vi "Router - Reader.vi"(8 "error in (no error)":errorcluster, 11 "Router Data In":T1) -> (0 "error out":errorcluster, 3 "Router Data Out":T1)   [LabVIEW 2016, in "PXImc Router.lvlib"]
uses:
  PXImc Router.lvlib
  Controls/Router - Configuration.ctl
  Controls/Target Type.ctl
  Controls/Router/Node Block R-W Properties.ctl
  Controls/Router/Block Properties.ctl
  Controls/Router/Router - PXImc Properties.ctl
  Controls/Router/Router - PXImc Card Properties.ctl
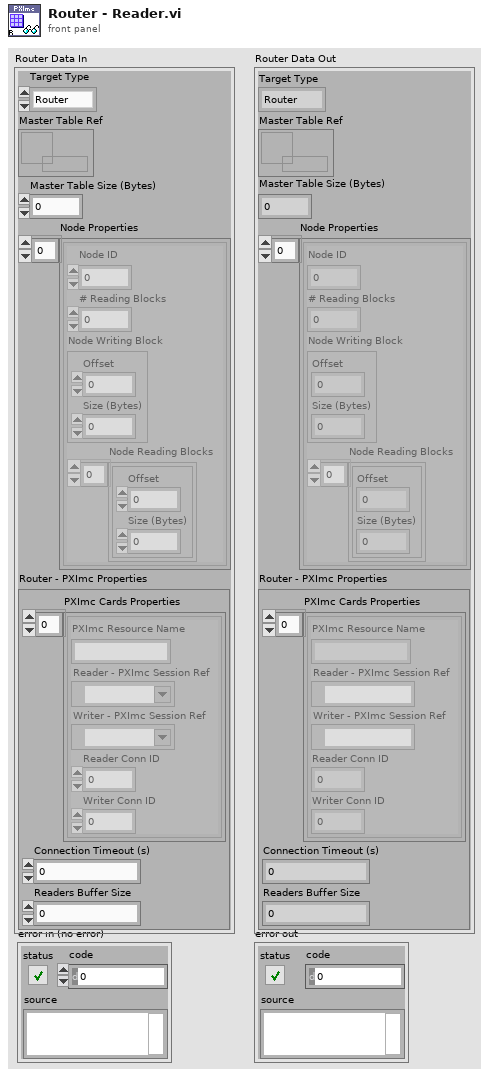
[diagram p1: front panel]
types:
  T1 = typedef "PXImc Router.lvlib/Router - Configuration.ctl" = cluster{"Target Type":T2, "Master Table Ref":refnum<data-value>, "Master Table Size (Bytes)":u32, "Node Properties":T3[], "Router - PXImc Properties":T5}
  T2 = typedef "PXImc Router.lvlib/Target Type.ctl" = enum16{"Router", "Node"}
  T3 = typedef "PXImc Router.lvlib/Node Block R-W Properties.ctl" = cluster{"Node ID":u32, "# Reading Blocks":u32, "Node Writing Block":T4, "Node Reading Blocks":T4[]}
  T4 = typedef "PXImc Router.lvlib/Block Properties.ctl" = cluster{"Offset":u32, "Size (Bytes)":u32}
  T5 = typedef "PXImc Router.lvlib/Router - PXImc Properties.ctl" = cluster{"PXImc Cards Properties":T6[], "Connection Timeout (s)":dbl, "Readers Buffer Size":u64}
  T6 = typedef "PXImc Router.lvlib/Router - PXImc Card Properties.ctl" = cluster{"PXImc Resource Name":string, "Reader - PXImc Session Ref":refnum<k21>, "Writer - PXImc Session Ref":refnum<k21>, "Reader Conn ID":u16, "Writer Conn ID":u16}
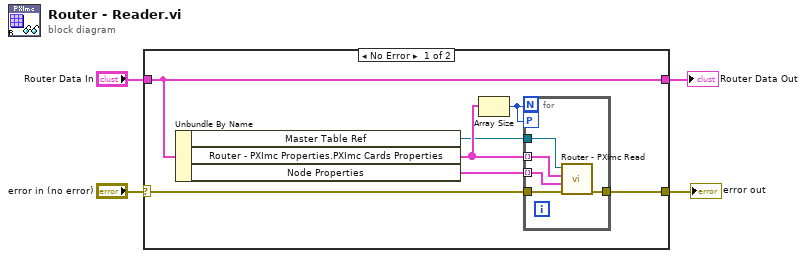
[diagram p0: block diagram]
diagram:
  n1 = case shown="No Error" "error in (no error)" {
    selector: "error in (no error)" -> [w11 w18]
    tunnel: [w5 w18] -> w3
    tunnel: "Router Data In" -> [w10 w17]
    tunnel: [w10 w17] -> w1
    frame No Error {
      n2 = Unbundle By Name(w10) -> ("Master Table Ref"=w6:refnum<data-value>, "Router - PXImc Properties.PXImc Cards Properties"=w8:T6[], "Node Properties"=w9:T3[])
      n3 = Array Size(array=w8) -> (size(s)=w7:i32)
      n4 = for {
        N: w7 -> [_]
        tunnel: w9 -> [w14] mode=indexing
        tunnel: w8 -> [w15] mode=indexing
        workers-P: w7 -> [_]
        tunnel: w11 -> [w13]
        tunnel: w6 -> [w16]
        tunnel: [w12] -> w5
        n5 = call "Router - PXImc Read.vi"("error in (no error)"=w13, "Node Properties"=w14, "PXImc Cards Properties"=w15, "Master Table Ref"=w16) -> ("error out"=w12:errorcluster)  [unwired: 7 in]
      }
    }
    frame Error {
    }
  }
  "error out" <- w3
  "Router Data Out" <- w1
